vi "Find HovaCAL N2 MFC.vi"() -> (3 "N2 MFC Idx":i32)   [LabVIEW 2020, in "Linearisierung v2.lvlib" / "Gasteiler.lvlib" / "HovaCAL_Interface.lvlib" / "Helper.lvlib"]
uses:
  Helper.lvlib
  Kommunikation/Aktion_FGV_HovaCAL_Interface_SetData.ctl
  Kommunikation/Kommunikation.lvlib
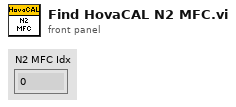
[diagram p1: front panel]
types:
  T1 = typedef "Linearisierung v2.lvlib/Gasteiler.lvlib/HovaCAL_Interface.lvlib/Kommunikation.lvlib/Aktion_FGV_HovaCAL_Interface_SetData.ctl" = enum16{"lesen", "Konzentrationen", "Pumpen Parameter", "Pumpe Konzentration", "Pumpe run", "Temperaturen", "Fluss", "Limits", "init"}
  T2 = cluster{"input concentration setpoint":dbl, "output concentration setpoint":dbl}[]
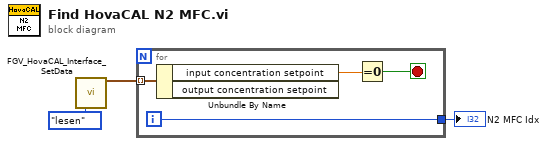
[diagram p0: block diagram]
diagram:
  n1 = call "FGV_HovaCAL_Interface_SetData.vi"("Aktion"=Aktion_FGV_HovaCAL_Interface_SetData."lesen") -> ("Set Values Cluster out"=w2:T2)  [unwired: 8 in, 6 out]
  n2 = for {
    tunnel: w2 -> [w7] mode=indexing
    tunnel: [w4] -> w1
    i -> [w4]
    stop <- w5 stop-if-true
    n3 = Unbundle By Name(w7) -> ("input concentration setpoint"=w6:dbl)  [unwired: 1 out]
    n4 = Equal To 0?(x=w6) -> (x = 0?=w5:bool)
  }
  "N2 MFC Idx" <- w1
